vi "S2C_GetRefs.vi"(8 "Error In":errorcluster, 10 "MenuRef":refnum<k9>, 11 "VI Ref":refnum<vi>) -> (0 "Error Out":errorcluster)   [LabVIEW 2015]
doc: "Aquires a reference to key front panel controls and stores the reference in a global."
uses:
  Globals/S2C_Globals.vi
  Globals/S2C_GlobalMenus.vi
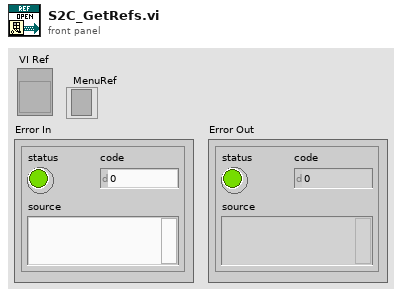
[diagram p1: front panel]
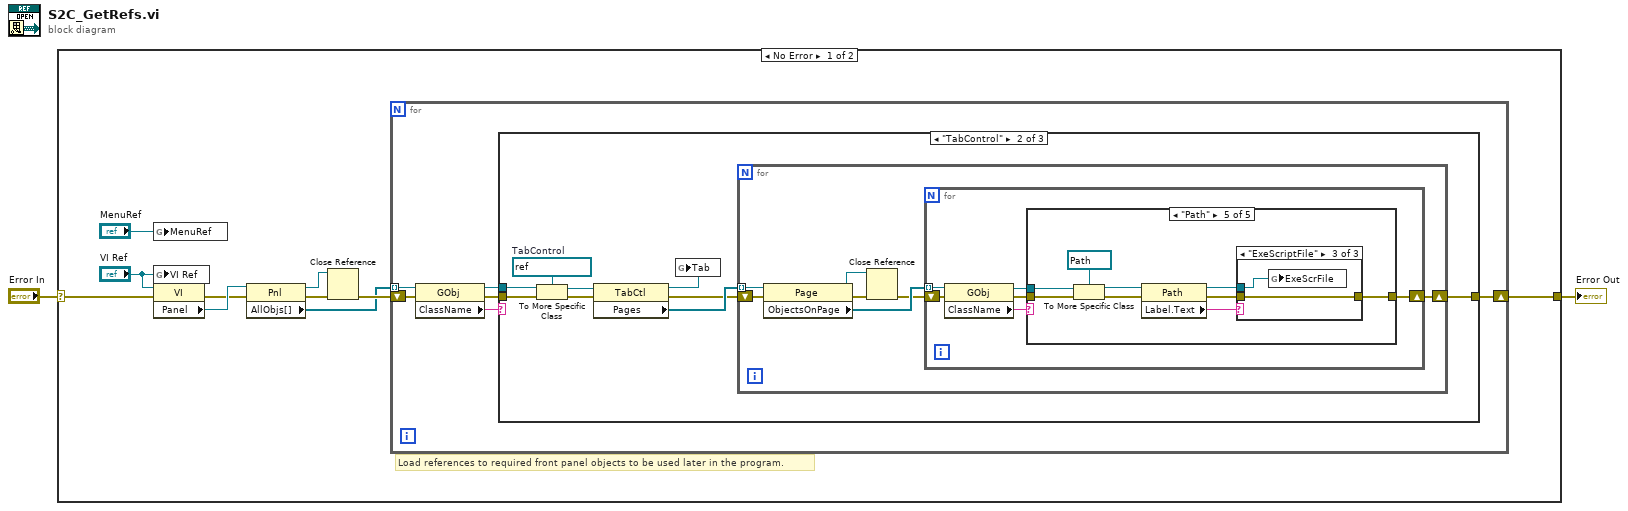
[diagram p0: block diagram]
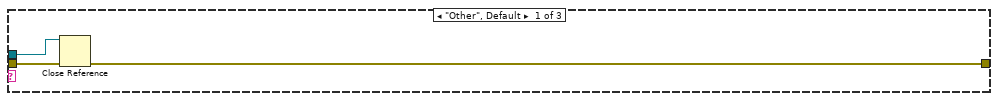
[diagram p2: hidden frame]
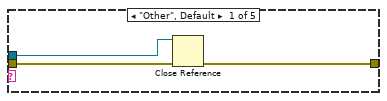
[diagram p3: hidden frame]
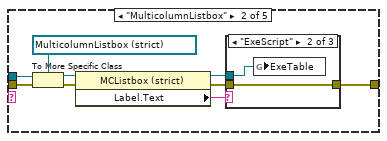
[diagram p4: hidden frame]
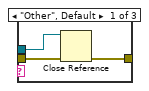
[diagram p5: hidden frame]
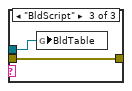
[diagram p6: hidden frame]
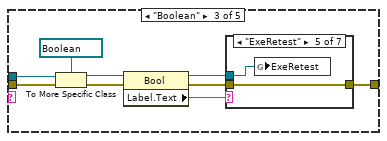
[diagram p7: hidden frame]
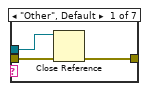
[diagram p8: hidden frame]
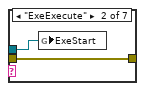
[diagram p9: hidden frame]
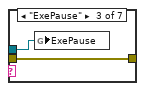
[diagram p10: hidden frame]
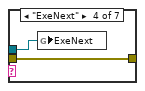
[diagram p11: hidden frame]
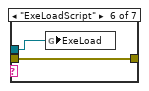
[diagram p12: hidden frame]
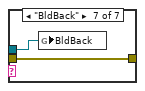
[diagram p13: hidden frame]
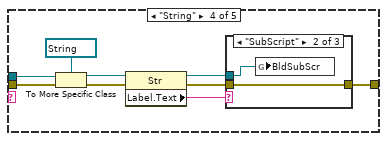
[diagram p14: hidden frame]
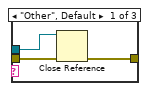
[diagram p15: hidden frame]
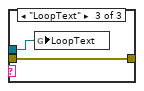
[diagram p16: hidden frame]
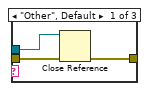
[diagram p17: hidden frame]
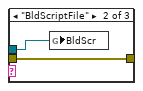
[diagram p18: hidden frame]
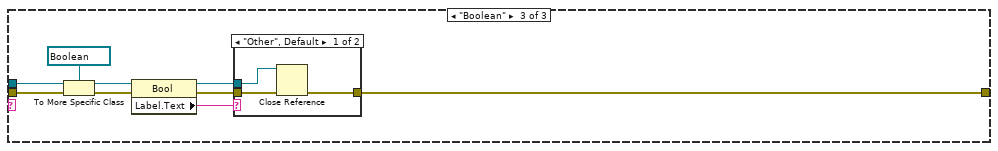
[diagram p19: hidden frame]
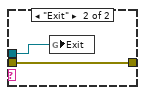
[diagram p20: hidden frame]
diagram:
  n1 = case shown="No Error" "Error In" {
    selector: "Error In" -> [w12 w133]
    tunnel: [w7 w133] -> w2
    frame No Error {
      # "Load references to required front panel objects to be used later in the program."
      n2 = global write "S2C_GlobalMenus.vi" "MenuRef"("MenuRef") -> ()
      n3 = global write "S2C_Globals.vi" "VI Ref"("VI Ref") -> ()
      n4 = property class="VI"(reference="VI Ref", error in=w12) -> (error out=w4:errorcluster, "Panel"=w5:refnum<vi>)  [unwired: 1 out]
      n5 = property class="Pnl"(reference=w5, error in=w4) -> (reference out=w10:refnum<vi>, error out=w11:errorcluster, "AllObjs[]"=w8:refnum<vi>[])
      n6 = Close Reference(reference=w10, error in (no error)=w11) -> (error out=w9:errorcluster)
      n7 = for {
        shift-right: [w13] -> w7
        shift-left: w9 -> [w17]
        tunnel: w8 -> [w18] mode=indexing
        n8 = property class="GObj"(reference=w18, error in=w17) -> (reference out=w14:refnum<vi>, error out=w16:errorcluster, "ClassName"=w15:string)
        n9 = case shown="\"TabControl\"" w15 {
          tunnel: w16 -> [w21 w30 w120]
          tunnel: w14 -> [w20 w25 w119]
          tunnel: [w19 w24 w127] -> w13
          frame "Other", Default {
            n10 = Close Reference(reference=w20, error in (no error)=w21) -> (error out=w19:errorcluster)
          }
          frame "TabControl" {
            w29 = refnum<vi> refnum  # TabControl
            n11 = To More Specific Class(target class=w29, reference=w25, error in=w30) -> (specific class reference=w28:refnum<vi>, error out=w27:errorcluster)
            n12 = property class="TabCtl"(reference=w28, error in=w27) -> (reference out=w22:refnum<vi>, error out=w23:errorcluster, "Pages"=w26:refnum<vi>[])
            n13 = global write "S2C_Globals.vi" "Tab"(w22) -> ()
            n14 = for {
              shift-right: [w31] -> w24
              shift-left: w23 -> [w36]
              tunnel: w26 -> [w37] mode=indexing
              n15 = property class="Page"(reference=w37, error in=w36) -> (reference out=w33:refnum<vi>, error out=w34:errorcluster, "ObjectsOnPage"=w35:refnum<vi>[])
              n16 = Close Reference(reference=w33, error in (no error)=w34) -> (error out=w32:errorcluster)
              n17 = for {
                tunnel: w35 -> [w42] mode=indexing
                shift-right: [w38] -> w31
                shift-left: w32 -> [w43]
                n18 = property class="GObj"(reference=w42, error in=w43) -> (reference out=w39:refnum<vi>, error out=w40:errorcluster, "ClassName"=w41:string)
                n19 = case shown="\"Path\"" w41 {
                  tunnel: w40 -> [w46 w55 w71 w95 w111]
                  tunnel: w39 -> [w45 w54 w70 w94 w110]
                  tunnel: [w44 w48 w64 w88 w104] -> w38
                  frame "Other", Default {
                    n20 = Close Reference(reference=w45, error in (no error)=w46) -> (error out=w44:errorcluster)
                  }
                  frame "MulticolumnListbox" {
                    n21 = To More Specific Class(target class=refnum<vi> refnum ("Exe_Ref"), reference=w54, error in=w55) -> (specific class reference=w52:refnum<vi>, error out=w53:errorcluster)
                    n22 = property class="MCListbox (strict)"(reference=w52, error in=w53) -> (reference out=w49:refnum<vi>, error out=w50:errorcluster, "Label.Text"=w51:string)
                    n23 = case shown="\"ExeScript\"" w51 {
                      tunnel: w50 -> [w58 w60 w62]
                      tunnel: w49 -> [w56 w59 w61]
                      tunnel: [w57 w60 w62] -> w48
                      frame "Other", Default {
                        n24 = Close Reference(reference=w56, error in (no error)=w58) -> (error out=w57:errorcluster)
                      }
                      frame "ExeScript" {
                        n25 = global write "S2C_Globals.vi" "ExeTable"(w59) -> ()
                      }
                      frame "BldScript" {
                        n26 = global write "S2C_Globals.vi" "BldTable"(w61) -> ()
                      }
                    }
                  }
                  frame "Boolean" {
                    n27 = To More Specific Class(target class=refnum<vi> refnum ("Execute"), reference=w70, error in=w71) -> (specific class reference=w68:refnum<vi>, error out=w69:errorcluster)
                    n28 = property class="Bool"(reference=w68, error in=w69) -> (reference out=w65:refnum<vi>, error out=w66:errorcluster, "Label.Text"=w67:string)
                    n29 = case shown="\"ExeRetest\"" w67 {
                      tunnel: w66 -> [w74 w76 w78 w80 w82 w84 w86]
                      tunnel: w65 -> [w72 w75 w77 w79 w81 w83 w85]
                      tunnel: [w73 w76 w78 w80 w82 w84 w86] -> w64
                      frame "Other", Default {
                        n30 = Close Reference(reference=w72, error in (no error)=w74) -> (error out=w73:errorcluster)
                      }
                      frame "ExeExecute" {
                        n31 = global write "S2C_Globals.vi" "ExeStart"(w75) -> ()
                      }
                      frame "ExePause" {
                        n32 = global write "S2C_Globals.vi" "ExePause"(w77) -> ()
                      }
                      frame "ExeNext" {
                        n33 = global write "S2C_Globals.vi" "ExeNext"(w79) -> ()
                      }
                      frame "ExeRetest" {
                        n34 = global write "S2C_Globals.vi" "ExeRetest"(w81) -> ()
                      }
                      frame "ExeLoadScript" {
                        n35 = global write "S2C_Globals.vi" "ExeLoad"(w83) -> ()
                      }
                      frame "BldBack" {
                        n36 = global write "S2C_Globals.vi" "BldBack"(w85) -> ()
                      }
                    }
                  }
                  frame "String" {
                    n37 = To More Specific Class(target class=refnum<vi> refnum ("Execute"), reference=w94, error in=w95) -> (specific class reference=w92:refnum<vi>, error out=w93:errorcluster)
                    n38 = property class="Str"(reference=w92, error in=w93) -> (reference out=w89:refnum<vi>, error out=w90:errorcluster, "Label.Text"=w91:string)
                    n39 = case shown="\"SubScript\"" w91 {
                      tunnel: w90 -> [w98 w100 w102]
                      tunnel: w89 -> [w96 w99 w101]
                      tunnel: [w97 w100 w102] -> w88
                      frame "Other", Default {
                        n40 = Close Reference(reference=w96, error in (no error)=w98) -> (error out=w97:errorcluster)
                      }
                      frame "SubScript" {
                        n41 = global write "S2C_Globals.vi" "BldSubScr"(w99) -> ()
                      }
                      frame "LoopText" {
                        n42 = global write "S2C_Globals.vi" "LoopText"(w101) -> ()
                      }
                    }
                  }
                  frame "Path" {
                    n43 = To More Specific Class(target class=refnum<vi> refnum ("Execute"), reference=w110, error in=w111) -> (specific class reference=w108:refnum<vi>, error out=w109:errorcluster)
                    n44 = property class="Path"(reference=w108, error in=w109) -> (reference out=w105:refnum<vi>, error out=w106:errorcluster, "Label.Text"=w107:string)
                    n45 = case shown="\"ExeScriptFile\"" w107 {
                      tunnel: w106 -> [w114 w116 w118]
                      tunnel: w105 -> [w112 w115 w117]
                      tunnel: [w113 w116 w118] -> w104
                      frame "Other", Default {
                        n46 = Close Reference(reference=w112, error in (no error)=w114) -> (error out=w113:errorcluster)
                      }
                      frame "BldScriptFile" {
                        n47 = global write "S2C_Globals.vi" "BldScr"(w115) -> ()
                      }
                      frame "ExeScriptFile" {
                        n48 = global write "S2C_Globals.vi" "ExeScrFile"(w117) -> ()
                      }
                    }
                  }
                }
              }
            }
          }
          frame "Boolean" {
            n49 = To More Specific Class(target class=refnum<vi> refnum ("Execute"), reference=w119, error in=w120) -> (specific class reference=w125:refnum<vi>, error out=w126:errorcluster)
            n50 = property class="Bool"(reference=w125, error in=w126) -> (reference out=w122:refnum<vi>, error out=w123:errorcluster, "Label.Text"=w124:string)
            n51 = case shown="\"Other\", Default" w124 {
              tunnel: w123 -> [w130 w132]
              tunnel: w122 -> [w128 w131]
              tunnel: [w129 w132] -> w127
              frame "Other", Default {
                n52 = Close Reference(reference=w128, error in (no error)=w130) -> (error out=w129:errorcluster)
              }
              frame "Exit" {
                n53 = global write "S2C_Globals.vi" "Exit"(w131) -> ()
              }
            }
          }
        }
      }
    }
    frame Error {
    }
  }
  "Error Out" <- w2
